vi "subStage_TrackTrajectory.vi"(7 "Track on?":bool, 8 "Stage Current Status":T1={" Current Position"=[-1.0, -12.0, 0.0], "Number of Axis"=3, "ILSID"=1}, 9 "Stage Previous Status":T1={" Current Position"=[-1.0, -12.0, 0.0], "Number of Axis"=3, "ILSID"=1}, 10 "Stage X Array In":dbl[](array[numeric]), 11 "Stage Y Array In":dbl[](array[numeric])) -> (2 "Stage X Array Out":dbl[](array[numeric]), 3 "Stage Y Array Out":dbl[](array[numeric]), 5 "Stage XY Cluster":cluster{dbl[], dbl[]})   [LabVIEW 2015]
panel:
  # "X"
  # "Y"
  # "X"
  # "Y"
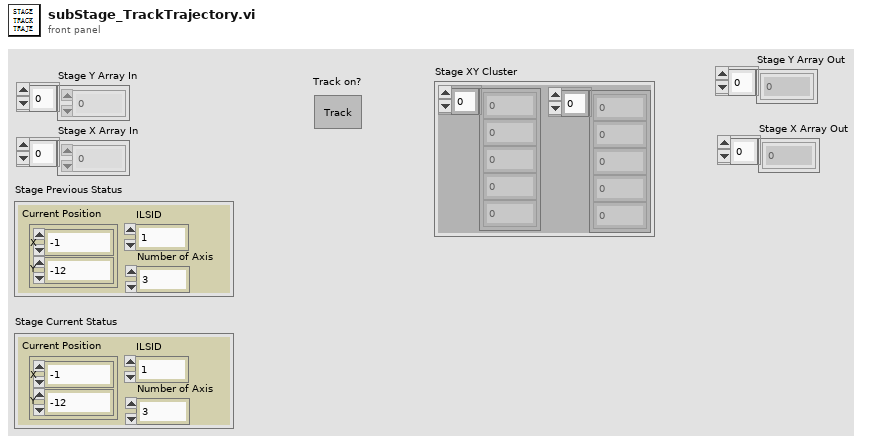
[diagram p1: front panel]
types:
  T1 = cluster{" Current Position":dbl[], "Number of Axis":i32, "ILSID":i32}
  T2 = cluster{"Stage Y Array In":dbl[], "Stage X Array In":dbl[]}
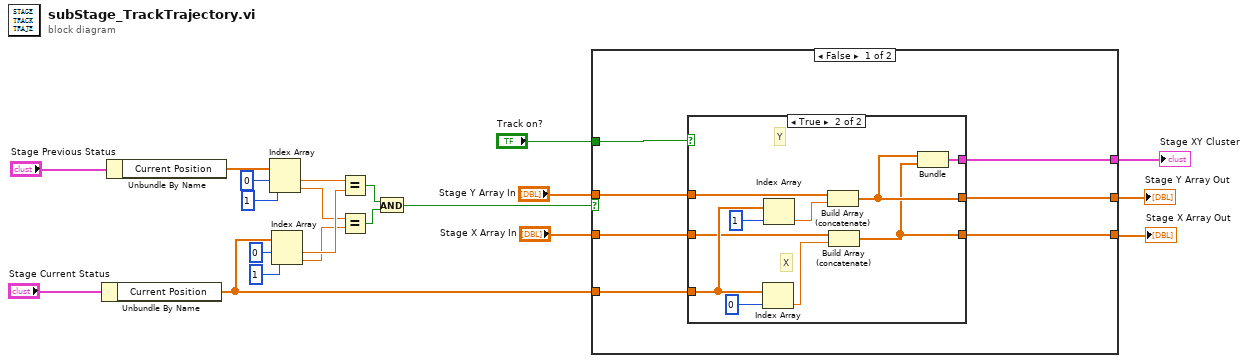
[diagram p0: block diagram]
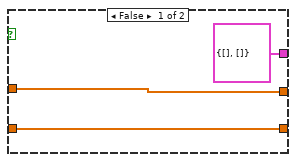
[diagram p2: hidden frame]
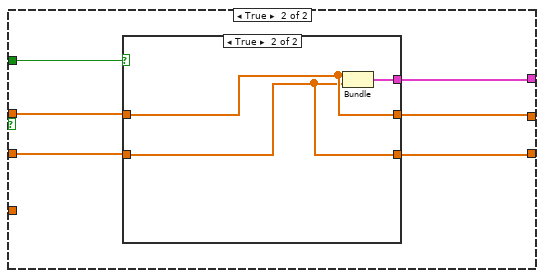
[diagram p3: hidden frame]
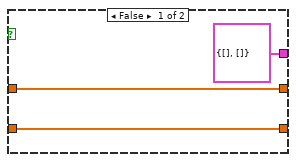
[diagram p4: hidden frame]
diagram:
  n1 = Unbundle By Name("Stage Current Status") -> ("Current Position"=w8:dbl[])
  n2 = Unbundle By Name("Stage Previous Status") -> ("Current Position"=w20:dbl[])
  n3 = Index Array(array=w20, index #1=0 ("index"), index #2=1 ("index")) -> (element #1=w15:dbl, element #2=w13:dbl)
  n4 = Index Array(array=w8, index #1=0 ("index"), index #2=1 ("index")) -> (element #1=w14:dbl, element #2=w12:dbl)
  n5 = Equal?(x=w15, y=w14) -> (x = y?=w10:bool)
  n6 = Equal?(x=w13, y=w12) -> (x = y?=w11:bool)
  n7 = And(x=w10, y=w11) -> (x .and. y?=w9:bool)
  n8 = case shown="False" w9 {
    tunnel: w8 -> [w28 _]
    tunnel: "Stage Y Array In" -> [w27 w46]
    tunnel: "Stage X Array In" -> [w26 w45]
    tunnel: [w25 w44] -> w4
    tunnel: [w24 w43] -> w3
    tunnel: "Track on?" -> [w23 w47]
    tunnel: [w22 w42] -> w1
    frame False {
      n9 = case shown="True" w23 {
        tunnel: w28 -> [_ w37]
        tunnel: [w30 w36] -> w25
        tunnel: [w29 w35] -> w24
        tunnel: [cluster{dbl[], dbl[]} {[], []} w34] -> w22
        tunnel: w26 -> [w29 w33]
        tunnel: w27 -> [w30 w32]
        frame False {
        }
        frame True {
          # "X"
          # "Y"
          n10 = Index Array(array=w37, index=0) -> (element=w40:dbl)
          n11 = Index Array(array=w37, index=1) -> (element=w39:dbl)
          n12 = Build Array (concatenate)(w32, w39) -> (w36:dbl[])
          n13 = Build Array (concatenate)(w33, w40) -> (w35:dbl[])
          n14 = Bundle(w36, w35) -> (w34:cluster{dbl[], dbl[]})  [unwired: 1 in]
        }
      }
    }
    frame True {
      n15 = case shown="True" w47 {
        tunnel: [cluster{dbl[], dbl[]} {[], []} w53] -> w42
        tunnel: w45 -> [w48 w51]
        tunnel: w46 -> [w49 w52]
        tunnel: [w49 w52] -> w44
        tunnel: [w48 w51] -> w43
        frame False {
        }
        frame True {
          n16 = Bundle("Stage Y Array In"=w52, "Stage X Array In"=w51) -> (w53:T2)  [unwired: 1 in]
        }
      }
    }
  }
  "Stage Y Array Out" <- w4
  "Stage X Array Out" <- w3
  "Stage XY Cluster" <- w1
